vi "写入多个寄存器 (子VI).vi"(8 "错误输入（无错误）":errorcluster, 9 "holding register value":u16 caption="保持寄存器值", 10 "address":u16 caption="地址", 11 "VISA resource name":refnum<visa-resource-name> caption="VISA资源名称") -> (0 "错误输出":errorcluster)   [LabVIEW 2016, in "斯坦道CODMn.lvlib"]
uses:
  <vilib>/NI/Modbus Library/API/Wrapper/Create Serial Master.vi
  <vilib>/NI/Modbus Library/API/master/Modbus Master.lvclass
  <vilib>/NI/Modbus Library/API/Wrapper/API Main.lvlib
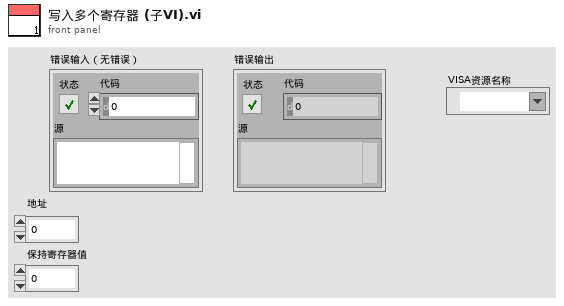
[diagram p1: front panel]
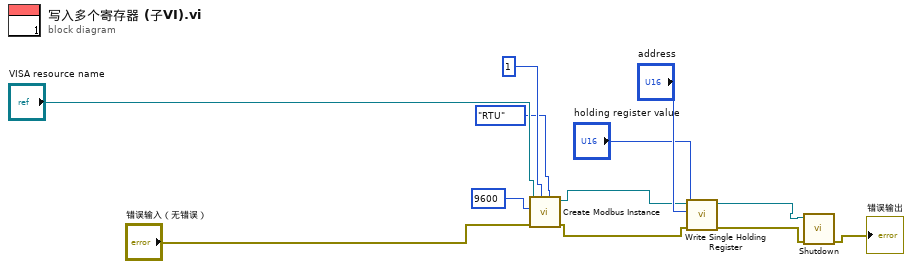
[diagram p0: block diagram]
diagram:
  n1 = call-poly <vilib>:"Create Modbus Instance.vi"("serial type"=enum16{"RTU", "ASCII"}."RTU", "unit ID"=u8 1, "error in"="错误输入（无错误）", "baud rate"=u32 9600 ("baud rate (9600)"), "VISA resource name"="VISA resource name") -> ("error out"=w4:errorcluster, "serial master instance"=w1:refnum<class "Modbus Master.lvclass">)  [unwired: 5 in]
  n2 = call-dynamic "Write Single Holding Register.vi"("error in"=w4, "register to write"="holding register value", "address"="address", "Modbus master in"=w1) -> ("error out"=w9:errorcluster, "Modbus master out"=w10:refnum<class "Modbus Master.lvclass">)  [unwired: 6 in]
  n3 = call-dynamic "Shutdown.vi"("error in"=w9, "Modbus master in"=w10) -> ("error out"=→"错误输出":errorcluster)  [unwired: 9 in]
